vi "CRYFlatten Text Open.vi"(11 "Flatten Data":string) -> (0 "bReslult":bool, 2 "Results Out":T1 {"Margin" format="%.2f"}, 3 "Curves Out":T3 {"Z data" items=["dB", "Lin"]; "X data" items=["dB", "Lin"]; "Y data" items=["dB", "Lin"]; "Z dB ref" format="%.1f"; "Z axis" items=["Log", "Lin"]; "X dB ref" format="%.1f"; "X axis" items=["Log", "Lin"]; "Y axis" items=["Log", "Lin"]; "Y dB ref" format="%.1f"; "Curve"."z" format="%.2f"; "Curve"."y" format="%.2f"; "Curve"."x" format="%.2f"})   [LabVIEW 2013]
uses:
  CRYSystem/Typedef Control/CRYData Cluster Array.ctl
  CRYSystem/Typedef Control/CRYData Cluster.ctl
  CRYSystem/Typedef Control/CRYResult Cluster Array.ctl
  CRYSystem/Typedef Control/CRYResult Cluster.ctl
panel:
  out "nPoint":i32
  out "Type":string
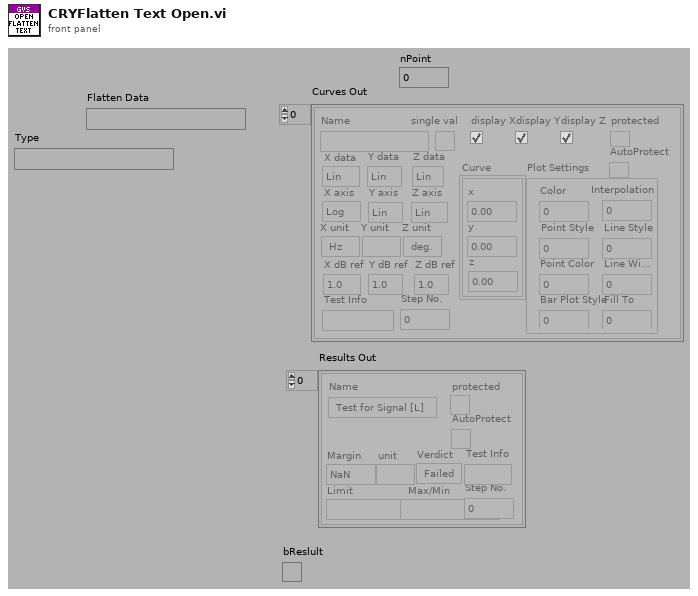
[diagram p1: front panel]
types:
  T1 = typedef "CRYResult Cluster Array.ctl" = T2[]
  T2 = typedef "CRYResult Cluster.ctl" = cluster{"Name":string, "Margin":dbl, "unit":string, "Verdict":bool, "Limit":string, "Max/Min":string, "protected":bool, "Step No.":i32, "Test Info":string, "AutoProtect":bool}
  T3 = typedef "CRYData Cluster Array.ctl" = T4[]
  T4 = typedef "CRYData Cluster.ctl" = cluster{"Name":string, "Curve":cluster{"x":dbl, "y":dbl, "z":dbl}[], "X data":u16, "Y data":u16, "Z data":u16, "X axis":u16, "Y axis":u16, "Z axis":u16, "X unit":string, "Y unit":string, "Z unit":string, "X dB ref":dbl, "Y dB ref":dbl, "Z dB ref":dbl, "single val":bool, "protected":bool, "display X":bool, "display Y":bool, "display Z":bool, "Test Info":string, "Step No.":i32, "Plot Settings":cluster{"Color":u32, "Interpolation":u8, "Point Style":u8, "Line Style":u8, "Point Color":u32, "Line Width":u8, "Bar Plot Style":u8, "Fill To":i16}, "AutoProtect":bool}
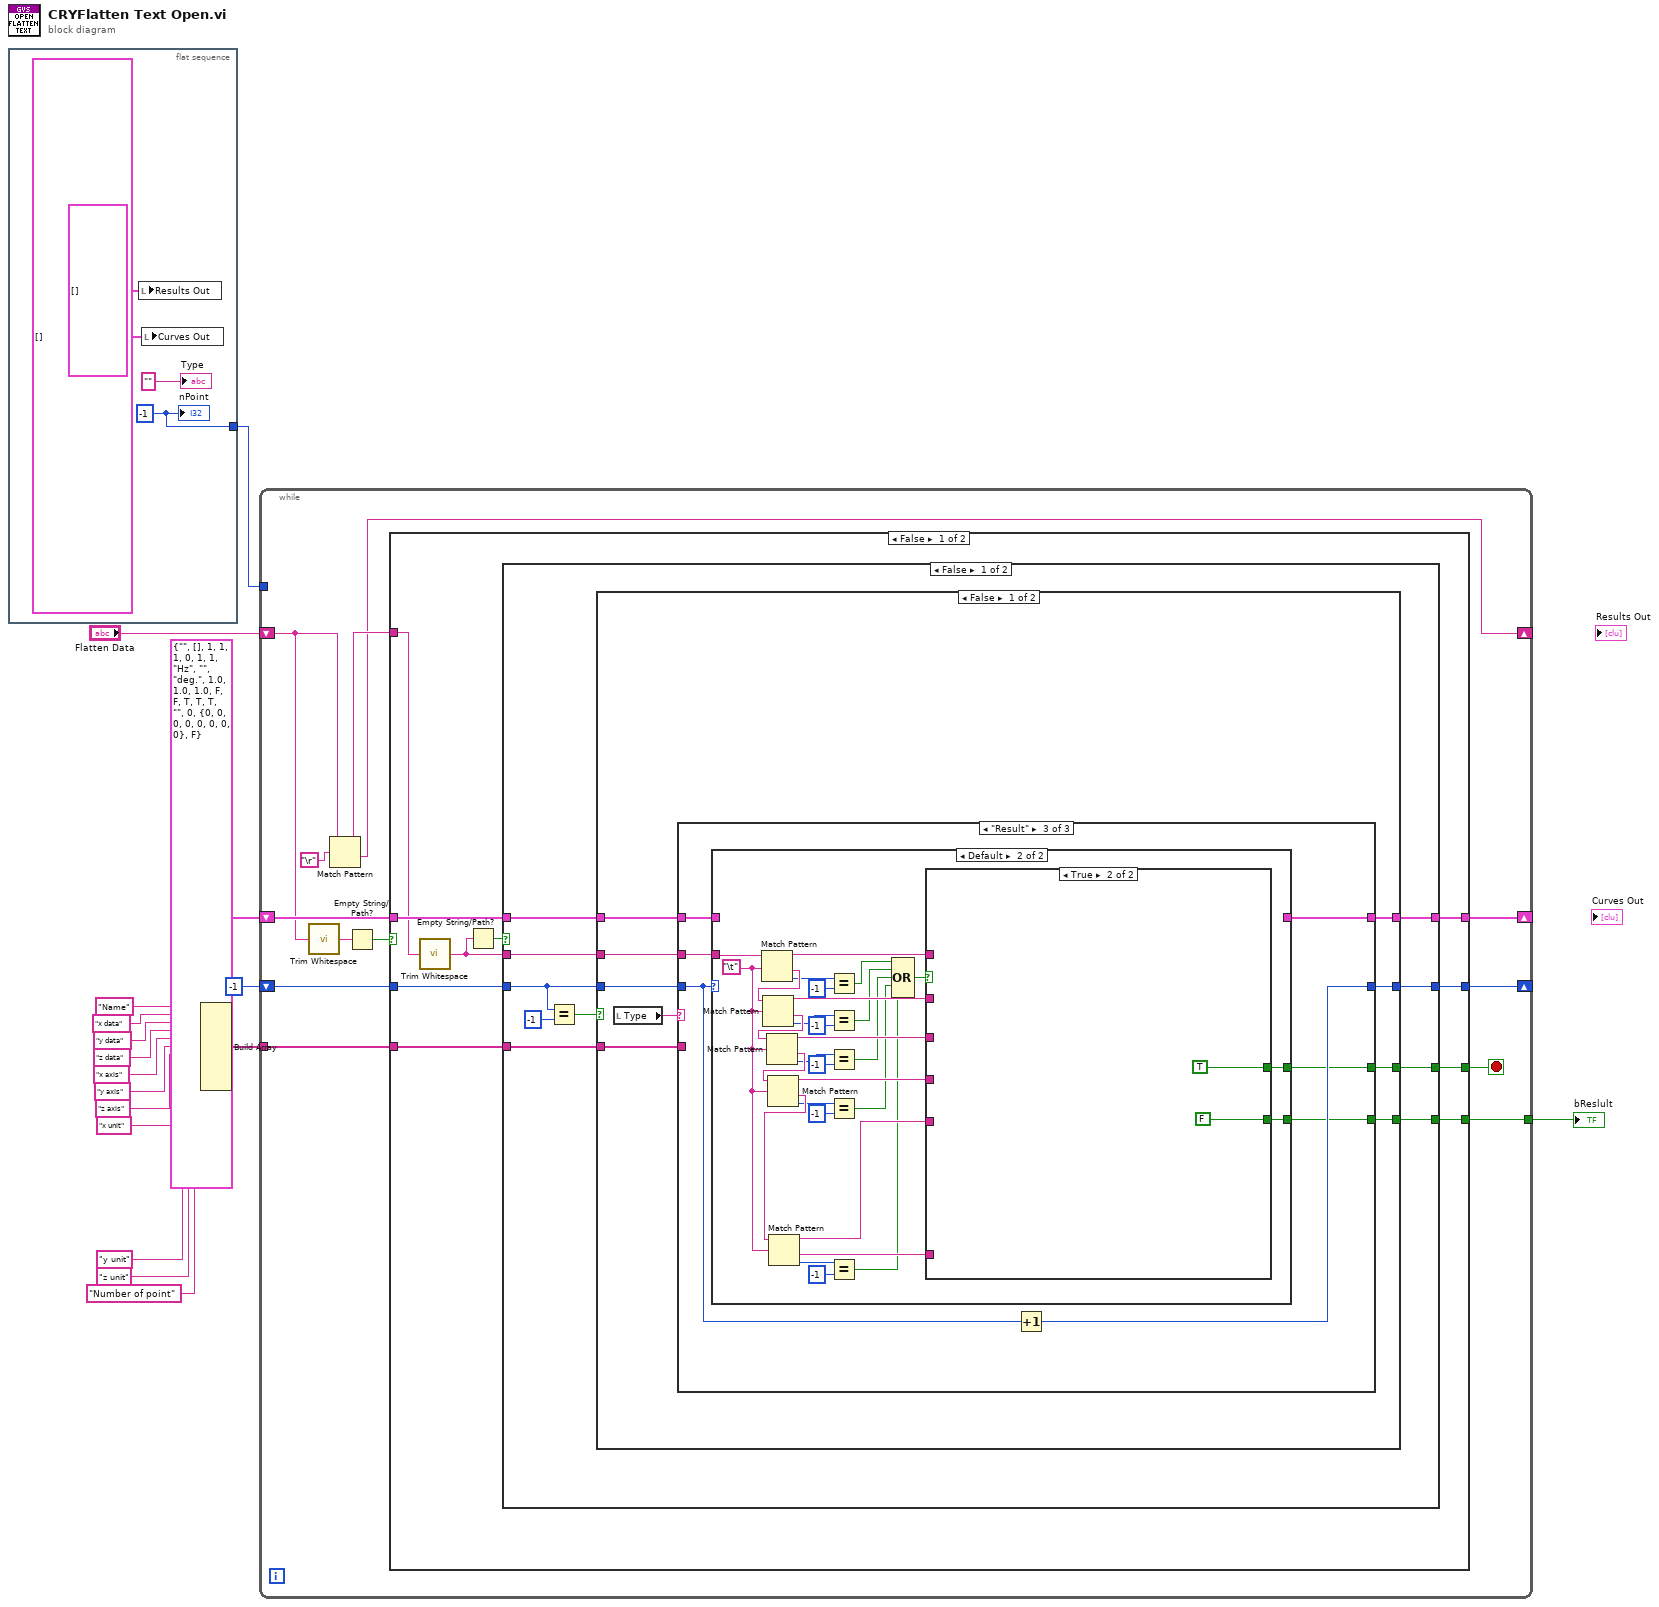
[diagram p0: block diagram]
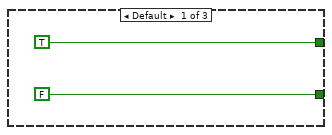
[diagram p2: hidden frame]
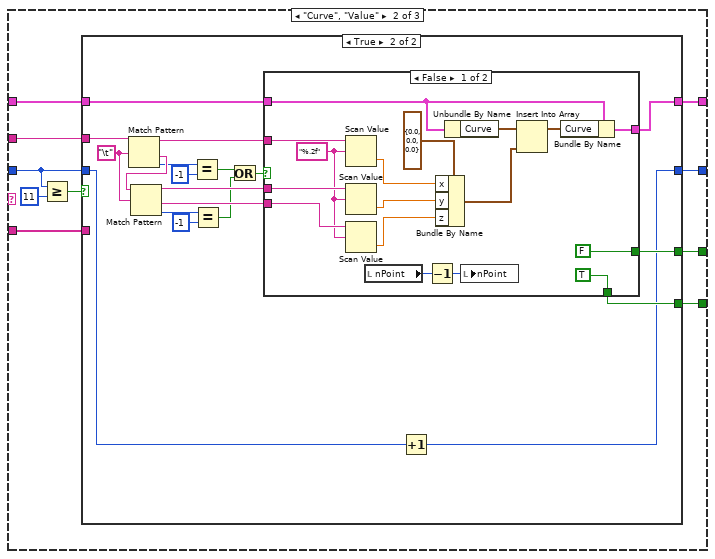
[diagram p3: hidden frame]
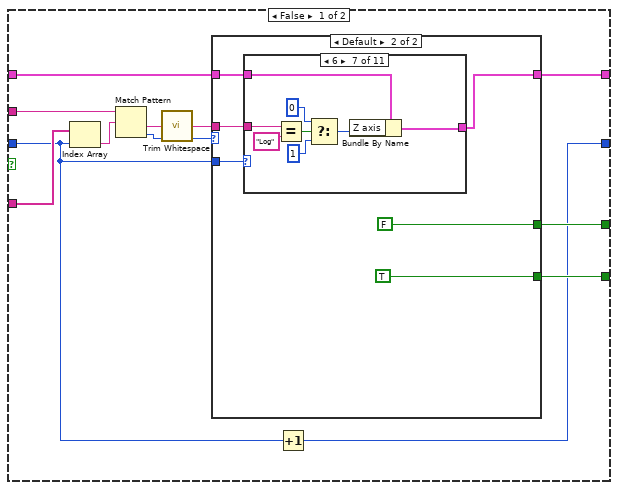
[diagram p4: hidden frame]
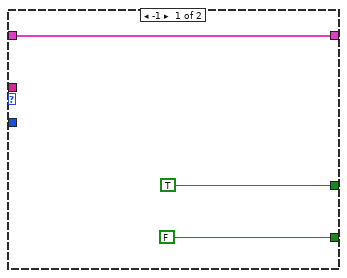
[diagram p5: hidden frame]
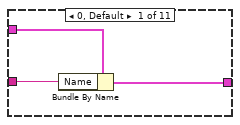
[diagram p6: hidden frame]
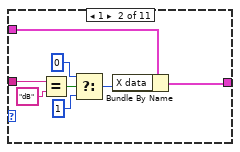
[diagram p7: hidden frame]
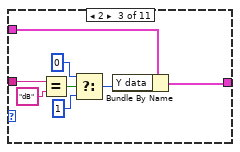
[diagram p8: hidden frame]
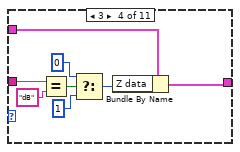
[diagram p9: hidden frame]
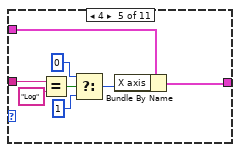
[diagram p10: hidden frame]
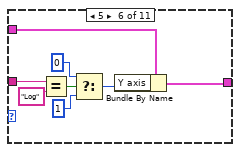
[diagram p11: hidden frame]
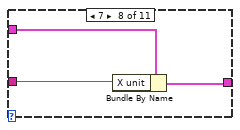
[diagram p12: hidden frame]
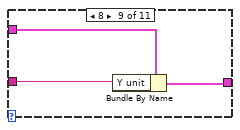
[diagram p13: hidden frame]
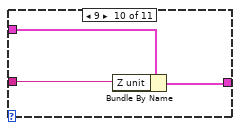
[diagram p14: hidden frame]
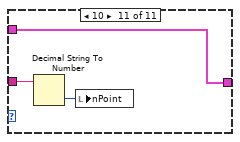
[diagram p15: hidden frame]
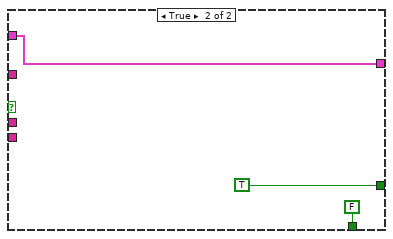
[diagram p16: hidden frame]
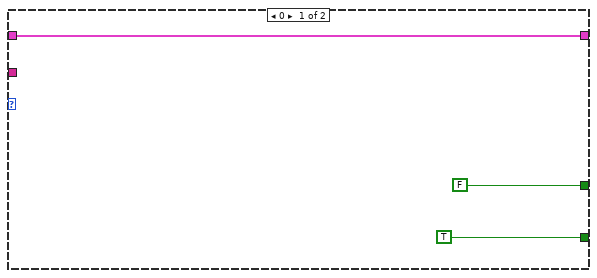
[diagram p17: hidden frame]
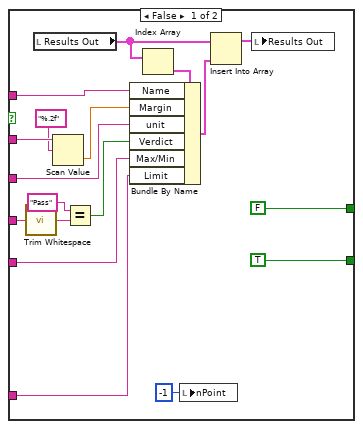
[diagram p18: hidden frame]
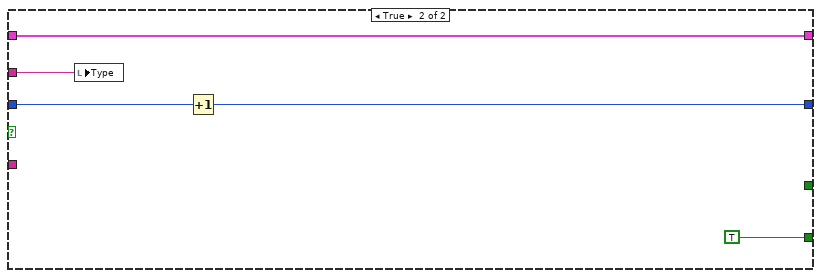
[diagram p19: hidden frame]
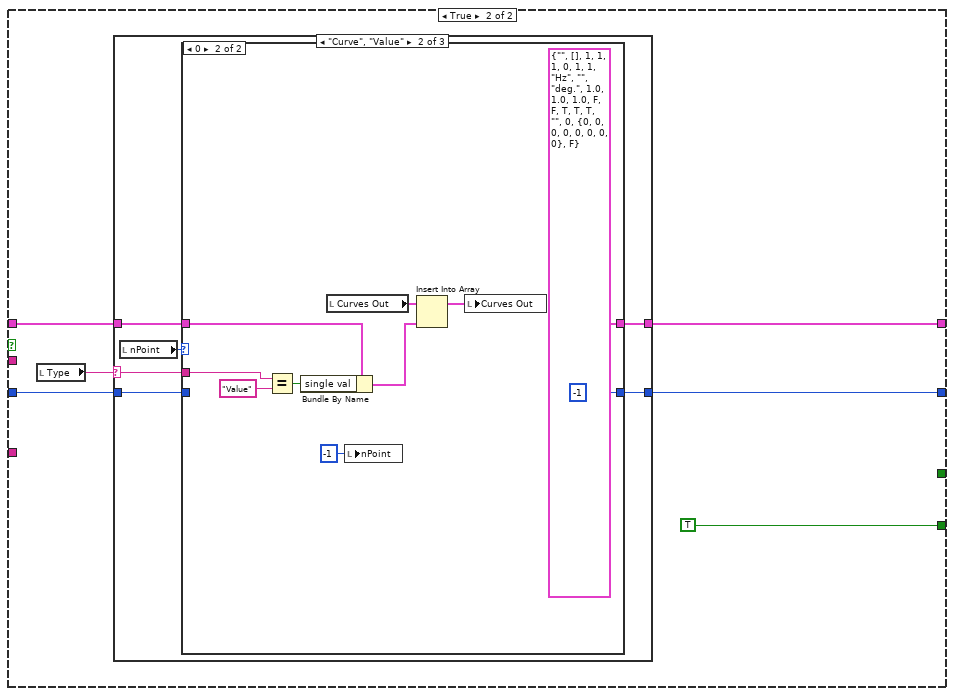
[diagram p20: hidden frame]
diagram:
  n1 = flat-sequence {
    tunnel: [w20] -> w1
    frame #0 {
      w20 = -1 ("nPoint")
      n2 = local write "Results Out"(T2[] []) -> ()
      n3 = local write "Curves Out"(T4[] []) -> ()
      "Type" <- "" ("Type")
      "nPoint" <- w20
    }
  }
  n4 = Build Array("Name", "x data", "y data", "z data", "x axis", "y axis", "z axis", "x unit", "y unit", "z unit", "Number of point") -> (w6:string[])
  n5 = while {
    shift-right: [w24] -> _
    shift-left: "Flatten Data" -> [w22]
    shift-right: [w32] -> _
    shift-left: T4 {"Name"="", "Curve"=[], "X data"=1, "Y data"=1, "Z data"=1, "X axis"=0, "Y axis"=1, "Z axis"=1, "X unit"="Hz", "Y unit"="", "Z unit"="deg.", "X dB ref"=1.0, "Y dB ref"=1.0, "Z dB ref"=1.0, "single val"=FALSE, "protected"=FALSE, "display X"=TRUE, "display Y"=TRUE, "display Z"=TRUE, "Test Info"="", "Step No."=0, "Plot Settings"={"Color"=0, "Interpolation"=0, "Point Style"=0, "Line Style"=0, "Point Color"=0, "Line Width"=0, "Bar Plot Style"=0, "Fill To"=0}, "AutoProtect"=FALSE} ("Curve") -> [w31]
    shift-right: [w25] -> _
    shift-left: -1 -> [w27]
    tunnel: w6 -> [w28]
    tunnel: [w26] -> w4
    tunnel: w1 -> [_]
    stop <- w30 stop-if-true
    n6 = call <vilib>:"Trim Whitespace.vi"("string"=w22) -> ("trimmed string"=w23:string)  [unwired: 1 in]
    n7 = Match Pattern(string=w22, regular expression="\r") -> (before substring=w33:string, after substring=w24:string)  [unwired: 1 in, 2 out]
    n8 = Empty String/Path?(string/path=w23) -> (empty?=w29:bool)
    n9 = case shown="False" w29 {
      tunnel: w33 -> [w42 _]
      tunnel: [w44 w294] -> w32
      tunnel: w31 -> [w43 w295]
      tunnel: [w35 w296] -> w30
      tunnel: w28 -> [w39 _]
      tunnel: w27 -> [w38 w292]
      tunnel: [w37 w296] -> w26
      tunnel: [w36 w293] -> w25
      frame False {
        n10 = call <vilib>:"Trim Whitespace.vi"("string"=w42) -> ("trimmed string"=w41:string)  [unwired: 1 in]
        n11 = Empty String/Path?(string/path=w41) -> (empty?=w40:bool)
        n12 = case shown="False" w40 {
          tunnel: [w54 w266] -> w44
          tunnel: w43 -> [w53 w267]
          tunnel: w41 -> [w47 _]
          tunnel: w39 -> [w52 _]
          tunnel: w38 -> [w48 w265]
          tunnel: [w51 TRUE ("bReslult")] -> w37
          tunnel: [w50 w268] -> w36
          tunnel: [w49 _] -> w35
          frame False {
            n13 = Equal?(x=w48, y=-1) -> (x = y?=w45:bool)
            n14 = case shown="False" w45 {
              tunnel: [w63 w262] -> w54
              tunnel: w53 -> [w62 w262]
              tunnel: w52 -> [w61 _]
              tunnel: [w60 TRUE ("bReslult")] -> w51
              tunnel: [w59 w259] -> w50
              tunnel: [w58 _] -> w49
              tunnel: w48 -> [w57 w260]
              tunnel: w47 -> [w56 w263]
              frame False {
                n15 = local read "Type"() -> (w55:string)
                n16 = case shown="\"Result\"" w55 {
                  tunnel: [_ w75 w202] -> w63
                  tunnel: w62 -> [_ w74 w203]
                  tunnel: w61 -> [_ w73 _]
                  tunnel: [FALSE ("bReslult") w72 w199] -> w60
                  tunnel: [_ w69 w204] -> w59
                  tunnel: [TRUE ("bReslult") w68 w200] -> w58
                  tunnel: w57 -> [_ w67 w205]
                  tunnel: w56 -> [_ w66 w201]
                  frame Default {
                  }
                  frame "Curve", "Value" {
                    n17 = Greater Or Equal?(x=w67, y=11) -> (x >= y?=w70:bool)
                    n18 = case shown="True" w70 {
                      tunnel: [w87 w168] -> w75
                      tunnel: w74 -> [w86 w178]
                      tunnel: w66 -> [w85 w177]
                      tunnel: w73 -> [w84 _]
                      tunnel: [w80 w163] -> w72
                      tunnel: w67 -> [w78 w162]
                      tunnel: [w77 w161] -> w69
                      tunnel: [w79 w164] -> w68
                      frame False {
                        n19 = Index Array(array=w84, index=w78) -> (element=w81:string)
                        n20 = Match Pattern(string=w85, regular expression=w81) -> (after substring=w83:string, offset past match=w82:i32)  [unwired: 1 in, 2 out]
                        n21 = call <vilib>:"Trim Whitespace.vi"("string"=w83) -> ("trimmed string"=w76:string)  [unwired: 1 in]
                        n22 = case shown="Default" w82 {
                          tunnel: [w90 w96] -> w87
                          tunnel: w86 -> [w90 w95]
                          tunnel: w76 -> [_ w94]
                          tunnel: w78 -> [_ w92]
                          tunnel: [FALSE ("bReslult") TRUE ("bReslult")] -> w80
                          tunnel: [TRUE ("bReslult") FALSE ("bReslult")] -> w79
                          frame -1 {
                          }
                          frame Default {
                            n23 = case shown="6" w92 {
                              tunnel: [w99 w106 w114 w122 w130 w138 w146 w149 w152 w155 w159] -> w96
                              tunnel: w95 -> [w98 w107 w115 w123 w131 w139 w147 w150 w153 w156 w159]
                              tunnel: w94 -> [w97 w100 w108 w116 w124 w132 w140 w148 w151 w154 w158]
                              frame 0, Default {
                                n24 = Bundle By Name(cluster=w98, "Name"=w97) -> (w99:T4)
                              }
                              frame 1 {
                                n25 = Equal?(x=w100, y="dB") -> (x = y?=w104:bool)
                                n26 = Select(t=u16 0 ("X data"), s=w104, f=u16 1 ("X data")) -> (s? t:f=w101:u16)
                                n27 = Bundle By Name(cluster=w107, "X data"=w101) -> (w106:T4)
                              }
                              frame 2 {
                                n28 = Equal?(x=w108, y="dB") -> (x = y?=w112:bool)
                                n29 = Select(t=u16 0 ("X data"), s=w112, f=u16 1 ("X data")) -> (s? t:f=w109:u16)
                                n30 = Bundle By Name(cluster=w115, "Y data"=w109) -> (w114:T4)
                              }
                              frame 3 {
                                n31 = Equal?(x=w116, y="dB") -> (x = y?=w120:bool)
                                n32 = Select(t=u16 0 ("X data"), s=w120, f=u16 1 ("X data")) -> (s? t:f=w117:u16)
                                n33 = Bundle By Name(cluster=w123, "Z data"=w117) -> (w122:T4)
                              }
                              frame 4 {
                                n34 = Equal?(x=w124, y="Log") -> (x = y?=w125:bool)
                                n35 = Select(t=u16 0 ("X data"), s=w125, f=u16 1 ("X data")) -> (s? t:f=w126:u16)
                                n36 = Bundle By Name(cluster=w131, "X axis"=w126) -> (w130:T4)
                              }
                              frame 5 {
                                n37 = Equal?(x=w132, y="Log") -> (x = y?=w136:bool)
                                n38 = Select(t=u16 0 ("X data"), s=w136, f=u16 1 ("X data")) -> (s? t:f=w133:u16)
                                n39 = Bundle By Name(cluster=w139, "Y axis"=w133) -> (w138:T4)
                              }
                              frame 6 {
                                n40 = Equal?(x=w140, y="Log") -> (x = y?=w144:bool)
                                n41 = Select(t=u16 0 ("X data"), s=w144, f=u16 1 ("X data")) -> (s? t:f=w141:u16)
                                n42 = Bundle By Name(cluster=w147, "Z axis"=w141) -> (w146:T4)
                              }
                              frame 7 {
                                n43 = Bundle By Name(cluster=w150, "X unit"=w148) -> (w149:T4)
                              }
                              frame 8 {
                                n44 = Bundle By Name(cluster=w153, "Y unit"=w151) -> (w152:T4)
                              }
                              frame 9 {
                                n45 = Bundle By Name(cluster=w156, "Z unit"=w154) -> (w155:T4)
                              }
                              frame 10 {
                                n46 = Decimal String To Number(string=w158) -> (number=w157:i32)  [unwired: 2 in, 1 out]
                                n47 = local write "nPoint"(w157) -> ()
                              }
                            }
                          }
                        }
                        n48 = Increment(x=w78) -> (x+1=w77:i32)
                      }
                      frame True {
                        w160 = "\t"
                        n49 = Match Pattern(string=w177, regular expression=w160) -> (before substring=w171:string, after substring=w176:string, offset past match=w175:i32)  [unwired: 1 in, 1 out]
                        n50 = Match Pattern(string=w176, regular expression=w160) -> (before substring=w170:string, after substring=w169:string, offset past match=w172:i32)  [unwired: 1 in, 1 out]
                        n51 = Equal?(x=w175, y=-1) -> (x = y?=w167:bool)
                        n52 = Equal?(x=w172, y=-1) -> (x = y?=w166:bool)
                        n53 = Or(x=w167, y=w166) -> (x .or. y?=w165:bool)
                        n54 = case shown="False" w165 {
                          tunnel: w178 -> [w195 w198]
                          tunnel: w171 -> [w190 _]
                          tunnel: w170 -> [w189 _]
                          tunnel: w169 -> [w188 _]
                          tunnel: [w183 w198] -> w168
                          tunnel: [FALSE ("bReslult") TRUE ("bReslult")] -> w164
                          tunnel: [TRUE ("bReslult") FALSE ("bReslult")] -> w163
                          frame False {
                            w187 = "%.2f" ("format string")
                            n55 = Scan Value(string=w190, format string=w187) -> (value=w186:dbl)  [unwired: 1 in, 1 out]
                            n56 = Scan Value(string=w189, format string=w187) -> (value=w185:dbl)  [unwired: 1 in, 1 out]
                            n57 = Scan Value(string=w188, format string=w187) -> (value=w184:dbl)  [unwired: 1 in, 1 out]
                            n58 = local read "nPoint"() -> (w180:i32)
                            n59 = Decrement(x=w180) -> (x-1=w181:i32)
                            n60 = Bundle By Name(cluster=cluster{"x":dbl, "y":dbl, "z":dbl} {"x"=0.0, "y"=0.0, "z"=0.0} ("new element/subarray"), "x"=w186, "y"=w185, "z"=w184) -> (w191:cluster{"x":dbl, "y":dbl, "z":dbl})
                            n61 = Unbundle By Name(w195) -> ("Curve"=w194:cluster{"x":dbl, "y":dbl, "z":dbl}[])
                            n62 = local write "nPoint"(w181) -> ()
                            n63 = Insert Into Array(array=w194, new element=w191) -> (w193:cluster{"x":dbl, "y":dbl, "z":dbl}[])  [unwired: 1 in]
                            n64 = Bundle By Name(cluster=w195, "Curve"=w193) -> (w183:T4)
                          }
                          frame True {
                          }
                        }
                        n65 = Increment(x=w162) -> (x+1=w161:i32)
                      }
                    }
                  }
                  frame "Result" {
                    n66 = case shown="Default" w205 {
                      tunnel: w203 -> [w208 _]
                      tunnel: [w208 _] -> w202
                      tunnel: w201 -> [_ w238]
                      tunnel: [FALSE w210] -> w200
                      tunnel: [TRUE w209] -> w199
                      frame 0 {
                      }
                      frame Default {
                        w234 = "\t"
                        n67 = Match Pattern(string=w238, regular expression=w234) -> (before substring=w233:string, after substring=w237:string, offset past match=w226:i32)  [unwired: 1 in, 1 out]
                        n68 = Match Pattern(string=w237, regular expression=w234) -> (before substring=w232:string, after substring=w235:string, offset past match=w217:i32)  [unwired: 1 in, 1 out]
                        n69 = Match Pattern(string=w235, regular expression=w234) -> (before substring=w231:string, after substring=w236:string, offset past match=w218:i32)  [unwired: 1 in, 1 out]
                        n70 = Match Pattern(string=w236, regular expression=w234) -> (before substring=w230:string, after substring=w220:string, offset past match=w219:i32)  [unwired: 1 in, 1 out]
                        n71 = Match Pattern(string=w220, regular expression=w234) -> (before substring=w229:string, after substring=w228:string, offset past match=w221:i32)  [unwired: 1 in, 1 out]
                        n72 = Equal?(x=w226, y=-1) -> (x = y?=w216:bool)
                        n73 = Equal?(x=w217, y=-1) -> (x = y?=w215:bool)
                        n74 = Equal?(x=w218, y=-1) -> (x = y?=w214:bool)
                        n75 = Equal?(x=w219, y=-1) -> (x = y?=w213:bool)
                        n76 = Equal?(x=w221, y=-1) -> (x = y?=w212:bool)
                        n77 = Compound Arithmetic op=OR(w216, w215, w214, w213, w212) -> (w211:bool)
                        n78 = case shown="True" w211 {
                          tunnel: w233 -> [w253 _]
                          tunnel: w232 -> [w252 _]
                          tunnel: w231 -> [w248 _]
                          tunnel: w230 -> [w247 _]
                          tunnel: w229 -> [w244 _]
                          tunnel: w228 -> [w243 _]
                          tunnel: [FALSE TRUE] -> w210
                          tunnel: [TRUE FALSE] -> w209
                          frame False {
                            n79 = call <vilib>:"Trim Whitespace.vi"("string"=w247) -> ("trimmed string"=w239:string)  [unwired: 1 in]
                            n80 = local read "Results Out"() -> (w255:T1)
                            n81 = Scan Value(string=w252, format string="%.2f") -> (value=w250:dbl)  [unwired: 1 in, 1 out]
                            n82 = Equal?(x="Pass", y=w239) -> (x = y?=w245:bool)
                            n83 = Index Array(array=w255) -> (element=w254:T2)  [unwired: 1 in]
                            n84 = Bundle By Name(cluster=w254, "Name"=w253, "Margin"=w250, "unit"=w248, "Verdict"=w245, "Max/Min"=w244, "Limit"=w243) -> (w249:T2)
                            n85 = local write "nPoint"(-1 ("nPoint")) -> ()
                            n86 = Insert Into Array(array=w255, new element=w249) -> (w256:T1)  [unwired: 1 in]
                            n87 = local write "Results Out"(w256) -> ()
                          }
                          frame True {
                          }
                        }
                      }
                    }
                    n88 = Increment(x=w205) -> (x+1=w204:i32)
                  }
                }
              }
              frame True {
                n89 = local write "Type"(w263) -> ()
                n90 = Increment(x=w260) -> (x+1=w259:i32)
              }
            }
          }
          frame True {
            n91 = local read "Type"() -> (w264:string)
            n92 = case shown="\"Curve\", \"Value\"" w264 {
              selector: w264 -> [_ w272 _]
              tunnel: [w271 w277 -1 ("y")] -> w268
              tunnel: w267 -> [w270 w276 _]
              tunnel: [w270 w275 _] -> w266
              tunnel: w265 -> [w271 w274 _]
              frame Default {
              }
              frame "Curve", "Value" {
                n93 = local read "nPoint"() -> (w273:i32)
                n94 = case shown="0" w273 {
                  tunnel: [w279 -1 ("y")] -> w277
                  tunnel: w274 -> [w279 _]
                  tunnel: w276 -> [w278 w281]
                  tunnel: [w278 T4 {"Name"="", "Curve"=[], "X data"=1, "Y data"=1, "Z data"=1, "X axis"=0, "Y axis"=1, "Z axis"=1, "X unit"="Hz", "Y unit"="", "Z unit"="deg.", "X dB ref"=1.0, "Y dB ref"=1.0, "Z dB ref"=1.0, "single val"=FALSE, "protected"=FALSE, "display X"=TRUE, "display Y"=TRUE, "display Z"=TRUE, "Test Info"="", "Step No."=0, "Plot Settings"={"Color"=0, "Interpolation"=0, "Point Style"=0, "Line Style"=0, "Point Color"=0, "Line Width"=0, "Bar Plot Style"=0, "Fill To"=0}, "AutoProtect"=FALSE} ("Curve")] -> w275
                  tunnel: w272 -> [_ w282]
                  frame Default {
                  }
                  frame 0 {
                    n95 = Equal?(x=w282, y="Value") -> (x = y?=w283:bool)
                    n96 = Bundle By Name(cluster=w281, "single val"=w283) -> (w280:T4)
                    n97 = local read "Curves Out"() -> (w287:T3)
                    n98 = local write "nPoint"(-1 ("nPoint")) -> ()
                    n99 = Insert Into Array(array=w287, new element=w280) -> (w288:T3)  [unwired: 1 in]
                    n100 = local write "Curves Out"(w288) -> ()
                  }
                }
              }
              frame "Result" {
              }
            }
          }
        }
      }
      frame True {
        w296 = TRUE
        n101 = local read "Type"() -> (w291:string)
        n102 = case shown="\"Curve\", \"Value\"" w291 {
          selector: w291 -> [_ w298 _]
          tunnel: w295 -> [_ w302 _]
          tunnel: [_ w301 _] -> w294
          tunnel: [w297 w300 -1 ("y")] -> w293
          tunnel: w292 -> [w297 w299 _]
          frame Default {
          }
          frame "Curve", "Value" {
            n103 = local read "nPoint"() -> (w303:i32)
            n104 = case shown="0" w303 {
              tunnel: [w305 -1 ("y")] -> w300
              tunnel: w299 -> [w305 _]
              tunnel: w302 -> [w304 w310]
              tunnel: [w304 T4 {"Name"="", "Curve"=[], "X data"=1, "Y data"=1, "Z data"=1, "X axis"=0, "Y axis"=1, "Z axis"=1, "X unit"="Hz", "Y unit"="", "Z unit"="deg.", "X dB ref"=1.0, "Y dB ref"=1.0, "Z dB ref"=1.0, "single val"=FALSE, "protected"=FALSE, "display X"=TRUE, "display Y"=TRUE, "display Z"=TRUE, "Test Info"="", "Step No."=0, "Plot Settings"={"Color"=0, "Interpolation"=0, "Point Style"=0, "Line Style"=0, "Point Color"=0, "Line Width"=0, "Bar Plot Style"=0, "Fill To"=0}, "AutoProtect"=FALSE} ("Curve")] -> w301
              tunnel: w298 -> [_ w306]
              frame Default {
              }
              frame 0 {
                n105 = Equal?(x=w306, y="Value") -> (x = y?=w307:bool)
                n106 = Bundle By Name(cluster=w310, "single val"=w307) -> (w309:T4)
                n107 = local read "Curves Out"() -> (w313:T3)
                n108 = local write "nPoint"(-1 ("nPoint")) -> ()
                n109 = Insert Into Array(array=w313, new element=w309) -> (w314:T3)  [unwired: 1 in]
                n110 = local write "Curves Out"(w314) -> ()
              }
            }
          }
          frame "Result" {
          }
        }
      }
    }
  }
  "bReslult" <- w4
